vi "Write Handle.vi"(8 "error in (no error)":errorcluster, 10 "Handle":u64, 11 "X509-Cert in":refnum<class "X509-Cert.lvclass">) -> (0 "error out":errorcluster, 3 "X509-Cert out":refnum<class "X509-Cert.lvclass">)   [LabVIEW 2013, in "SSL_Lib.lvlib" / "X509-Cert.lvclass"]
uses:
  X509-Cert.lvclass
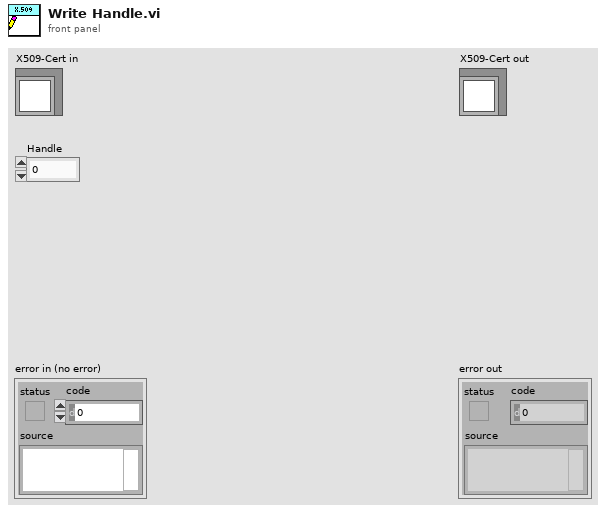
[diagram p1: front panel]
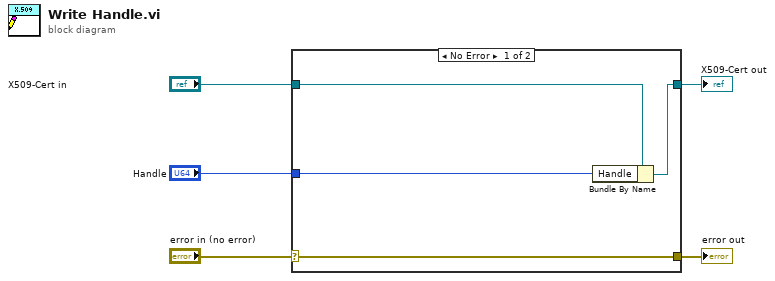
[diagram p0: block diagram]
diagram:
  n1 = case shown="No Error" "error in (no error)" {
    selector: "error in (no error)" -> [w9 w10]
    tunnel: [w9 w10] -> w4
    tunnel: [w7 w11] -> w2
    tunnel: "X509-Cert in" -> [w8 w11]
    tunnel: "Handle" -> [w6 _]
    frame No Error {
      n2 = Bundle By Name(cluster=w8, "Handle"=w6) -> (w7:refnum<class "X509-Cert.lvclass">)
    }
    frame Error {
    }
  }
  "error out" <- w4
  "X509-Cert out" <- w2
